vi "Describe Comparison.vi"(8 "error in (no error)":errorcluster, 9 "Control Value 2":variant, 10 "Control Value 1":variant) -> (0 "error out":errorcluster, 2 "Description":string)   [LabVIEW 2020, in "Identical Inputs Comparator.lvclass"]
uses:
  Identical Inputs Comparator.lvclass
  Identical Inputs Comparator.lvclass/Identical Inputs Comparator.ctl
  Core/Comparator/Comparator.lvclass
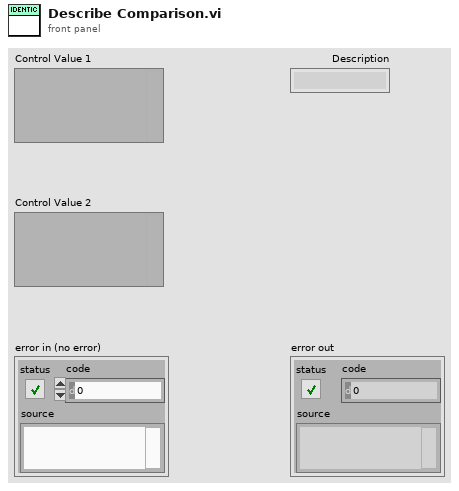
[diagram p1: front panel]
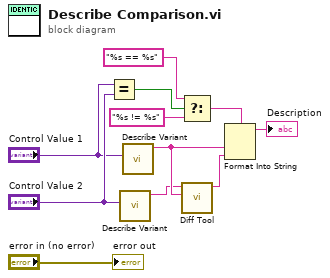
[diagram p0: block diagram]
diagram:
  n1 = Equal?(x="Control Value 1", y="Control Value 2") -> (x = y?=w3:bool)
  n2 = call "Describe Variant.vi"("Variant"="Control Value 2") -> ("Description with Type"=w6:string)  [unwired: 8 in, 2 out]
  n3 = call "Describe Variant.vi"("Variant"="Control Value 1") -> ("Description with Type"=w7:string)  [unwired: 8 in, 2 out]
  n4 = Select(t="%s == %s", s=w3, f="%s != %s") -> (s? t:f=w9:string)
  n5 = call "Diff Tool.vi"("Reference"=w7, "Target"=w6) -> ("Result"=w4:string)  [unwired: 8 in, 1 out]
  n6 = Format Into String(format string=w9, w7, w4) -> (resulting string=→"Description":string)  [unwired: 2 in, 1 out]
  "error out" <- "error in (no error)"
